vi "Moving_Average.vi"(1 "Period":i32=1, 2 "Input Array":dbl[](array[numeric])) -> (0 "N+1-Period":dbl[](graph))   [LabVIEW 2011]
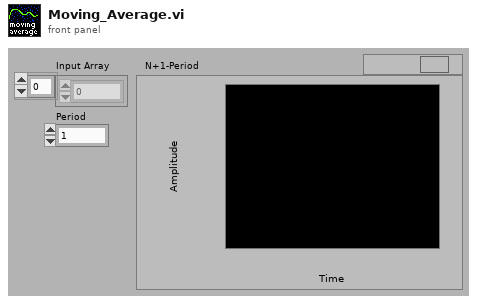
[diagram p1: front panel]
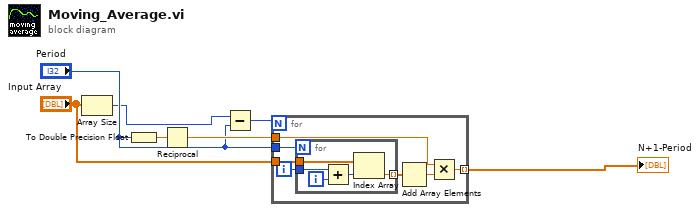
[diagram p0: block diagram]
diagram:
  n1 = Array Size(array="Input Array") -> (size(s)=w3:i32)
  n2 = To Double Precision Float(number="Period") -> (double precision float=w5:dbl)
  n3 = Reciprocal(x=w5) -> (1/x=w6:dbl)
  n4 = Subtract(x=w3, y="Period") -> (x-y=w1:i32)
  n5 = for {
    N: w1 -> [_]
    tunnel: "Period" -> [w14]
    tunnel: "Input Array" -> [w12]
    tunnel: w6 -> [w11]
    tunnel: [w8] -> w2 mode=indexing
    i -> [w13]
    n6 = for {
      N: w14 -> [_]
      tunnel: w13 -> [w19]
      tunnel: w12 -> [w16]
      tunnel: [w15] -> w9 mode=indexing
      i -> [w18]
      n7 = Add(x=w19, y=w18) -> (x+y=w17:i32)
      n8 = Index Array(array=w16, index=w17) -> (element=w15:dbl)
    }
    n9 = Add Array Elements(numeric array=w9) -> (sum=w10:dbl)
    n10 = Multiply(x=w11, y=w10) -> (x*y=w8:dbl)
  }
  "N+1-Period" <- w2
